vi "Generate Signal.vi"(0 "task in":refnum<k21>, 1 "Signal Spec":T1={"Duration"=0, "Intensity"=100, "Rate"=10} {"Rate" min=1 max=1000 step=1 format="%d Hz"; "Intensity" min=1 max=500 step=1 format="%d mV"; "Duration" min=1 max=5 step=1 format="%d ms"}, 2 "Timer":cluster{"Repeat?":bool, "Timer":u32} {"Timer" min=1 max=5 step=1 format="%d s"}, 11 "error in (no error)":errorcluster) -> (4 "task out":refnum<k21>, 6 "Scan Rate (Hz)":dbl, 8 "Data":dbl[](array[numeric]), 15 "error out":errorcluster)   [LabVIEW 2014]
uses:
  <vilib>/measure/NI_MABase.lvlib
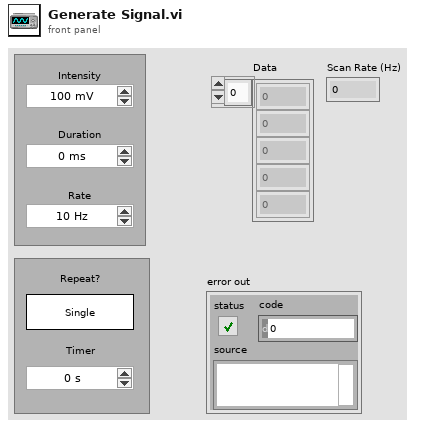
[diagram p1: front panel]
types:
  T1 = cluster{"Duration":u16, "Intensity":u16, "Rate":u16}
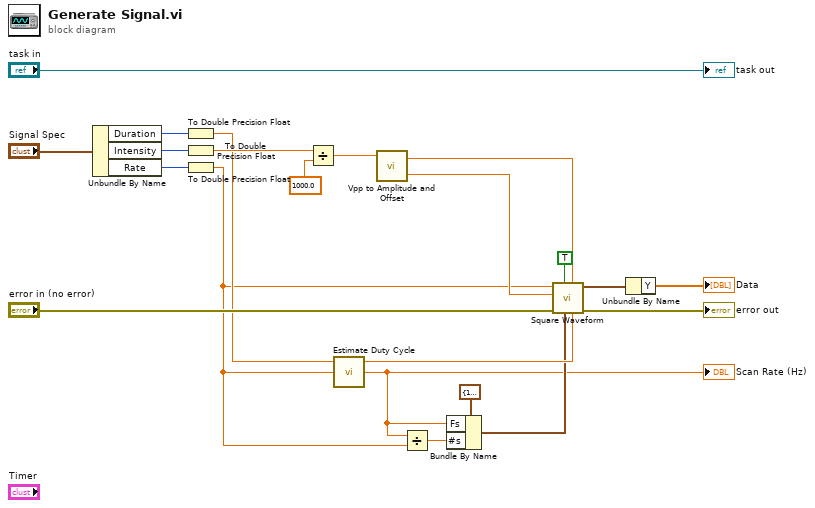
[diagram p0: block diagram]
diagram:
  n1 = Unbundle By Name("Signal Spec") -> ("Duration"=w19:u16, "Intensity"=w21:u16, "Rate"=w20:u16)
  n2 = To Double Precision Float(number=w19) -> (double precision float=w6:dbl)
  n3 = To Double Precision Float(number=w21) -> (double precision float=w8:dbl)
  n4 = To Double Precision Float(number=w20) -> (double precision float=w2:dbl)
  n5 = Divide(x=w8, y=1000.0) -> (x/y=w9:dbl)
  n6 = call "Estimate Duty Cycle.vi"("Rate (Hz)"=w2, "Duration (ms)"=w6) -> ("Scan Rate (Hz)"=w3:dbl, "Duty Cycle (%)"=w10:dbl)  [unwired: 2 in]
  "Scan Rate (Hz)" <- w3
  n7 = call "Vpp to Amplitude and Offset.vi"("Vpp"=w9) -> ("Amplitude"=w15:dbl, "Offset"=w14:dbl)  [unwired: 3 in]
  n8 = Divide(x=w3, y=w2) -> (x/y=w1:dbl)
  n9 = Bundle By Name(cluster=cluster{"Fs":dbl, "#s":dbl} {"Fs"=1000.0, "#s"=1000.0} ("sampling info"), "Fs"=w3, "#s"=w1) -> (w4:cluster{"Fs":dbl, "#s":dbl})
  n10 = call <vilib>:"Square Waveform.vi"("duty cycle (%)"=w10, "offset"=w14, "sampling info"=w4, "reset signal"=TRUE, "error in (no error)"="error in (no error)", "amplitude"=w15, "frequency"=w2) -> ("error out"=→"error out":errorcluster, "signal out"=w12:waveform(dbl))  [unwired: 3 in]
  n11 = Unbundle By Name(w12) -> ("Y"=→"Data":dbl[])
  "task out" <- "task in"
